vi "dynamic_lights.vi"() -> ()   [LabVIEW 2025]
uses:
  <vilib>/MakerHub/LINX/Public/Peripherals/Digital/Digital Write 1 Chan.vi
  <vilib>/MakerHub/LINX/Public/Peripherals/Digital/Digital Write N Chans.vi
  <vilib>/MakerHub/LINX/Private/Local IO/LinxDigitalWrite.vi
  <vilib>/MakerHub/LINX/Public/Utilities/Check Channel.vi
  <vilib>/MakerHub/LINX/Private/Utilties/Generate Error.vi
  <vilib>/Utility/file.llb/Read Delimited Spreadsheet (DBL).vi
  <vilib>/MakerHub/LINX/Public/Utilities/Open Serial.vi
  <vilib>/MakerHub/LINX/LMH-LINX.lvlib
panel:
  in  "em 2":bool
  in  "em 1":bool
  out "Emergency 2":bool
  out "Emergency 1":bool
  in  "Stop Button":bool
  in  "Stop":bool
  out "Lane 1 Elapsed Time":dbl
  out "Red 2":bool
  out "Orange 2":bool
  out "Green 2":bool
  out "Red 1":bool
  out "Orange 1":bool
  out "Green 1":bool
  out "Lan 2 Elapsed Time":dbl
  out "Lane 2 PCE":dbl
  out "Lane 1 PCE":dbl
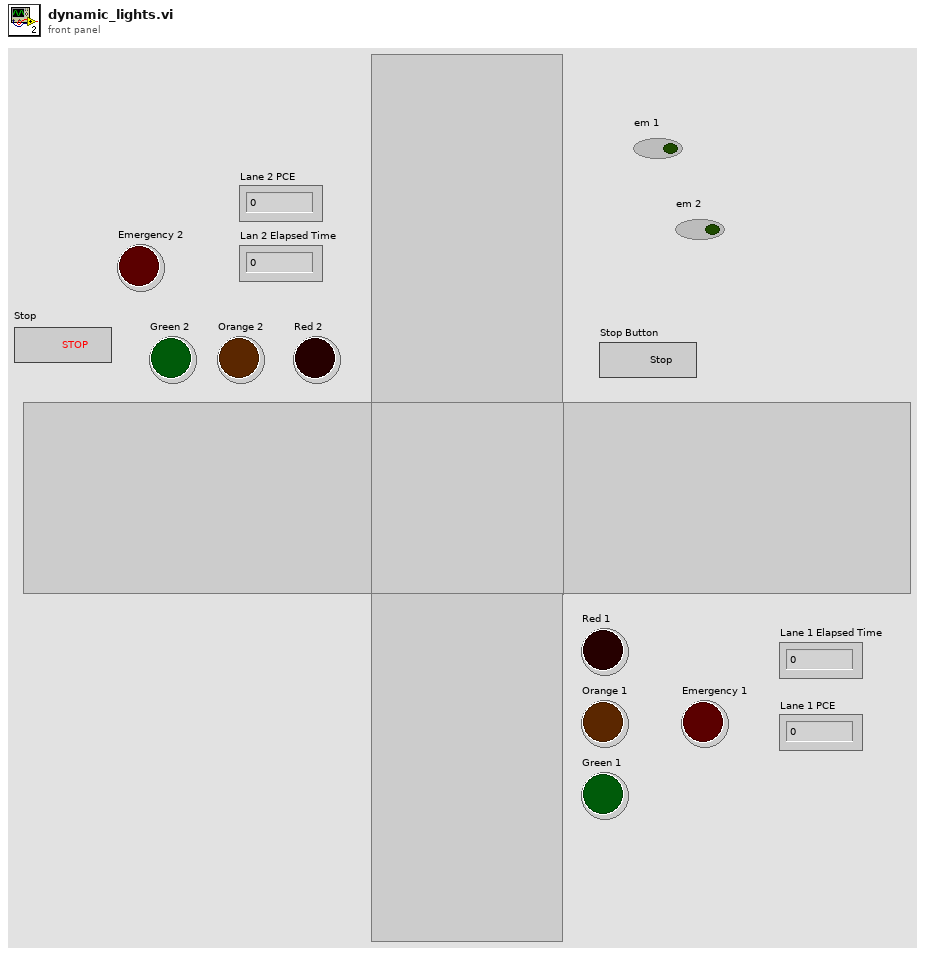
[diagram p1: front panel]
types:
  T1 = typedef "LMH-LINX.lvlib/LINX Ref.ctl" = cluster{"IO":T2, "Interface":T3, "LINX Device Config":T4}
  T2 = typedef "LMH-LINX.lvlib/Platform.ctl" = enum16{"Remote", "Local"}
  T3 = typedef "LMH-LINX.lvlib/Interface.ctl" = enum16{"Serial", "TCP"}
  T4 = typedef "LMH-LINX.lvlib/Device.lvlib/LINX Device Config.ctl" = cluster{"Interface":T3, "COM Port":refnum<visa-resource-name>, "TCP Configuration":T5, "Device Family":u8, "Device ID":u8, "Device Name":string, "TCP Ref":refnum<k5>, "Channels":T6}
  T5 = typedef "LMH-LINX.lvlib/Device.lvlib/TCP Config.ctl" = cluster{"IP Address":string, "Port":u16}
  T6 = typedef "LMH-LINX.lvlib/Channels.ctl" = cluster{"DI":u8[], "DO":u8[], "AI":u8[], "AO":u8[], "PWM":u8[], "QE":u8[], "UART":u8[], "I2C 2":u8[], "SPI":u8[], "CAN":u8[], "Servo":u8[], "AI Ref (V)":dbl, "AI Resolution (Bits)":u8, "AO Ref (V)":dbl, "AO Resolution (Bits)":u8}
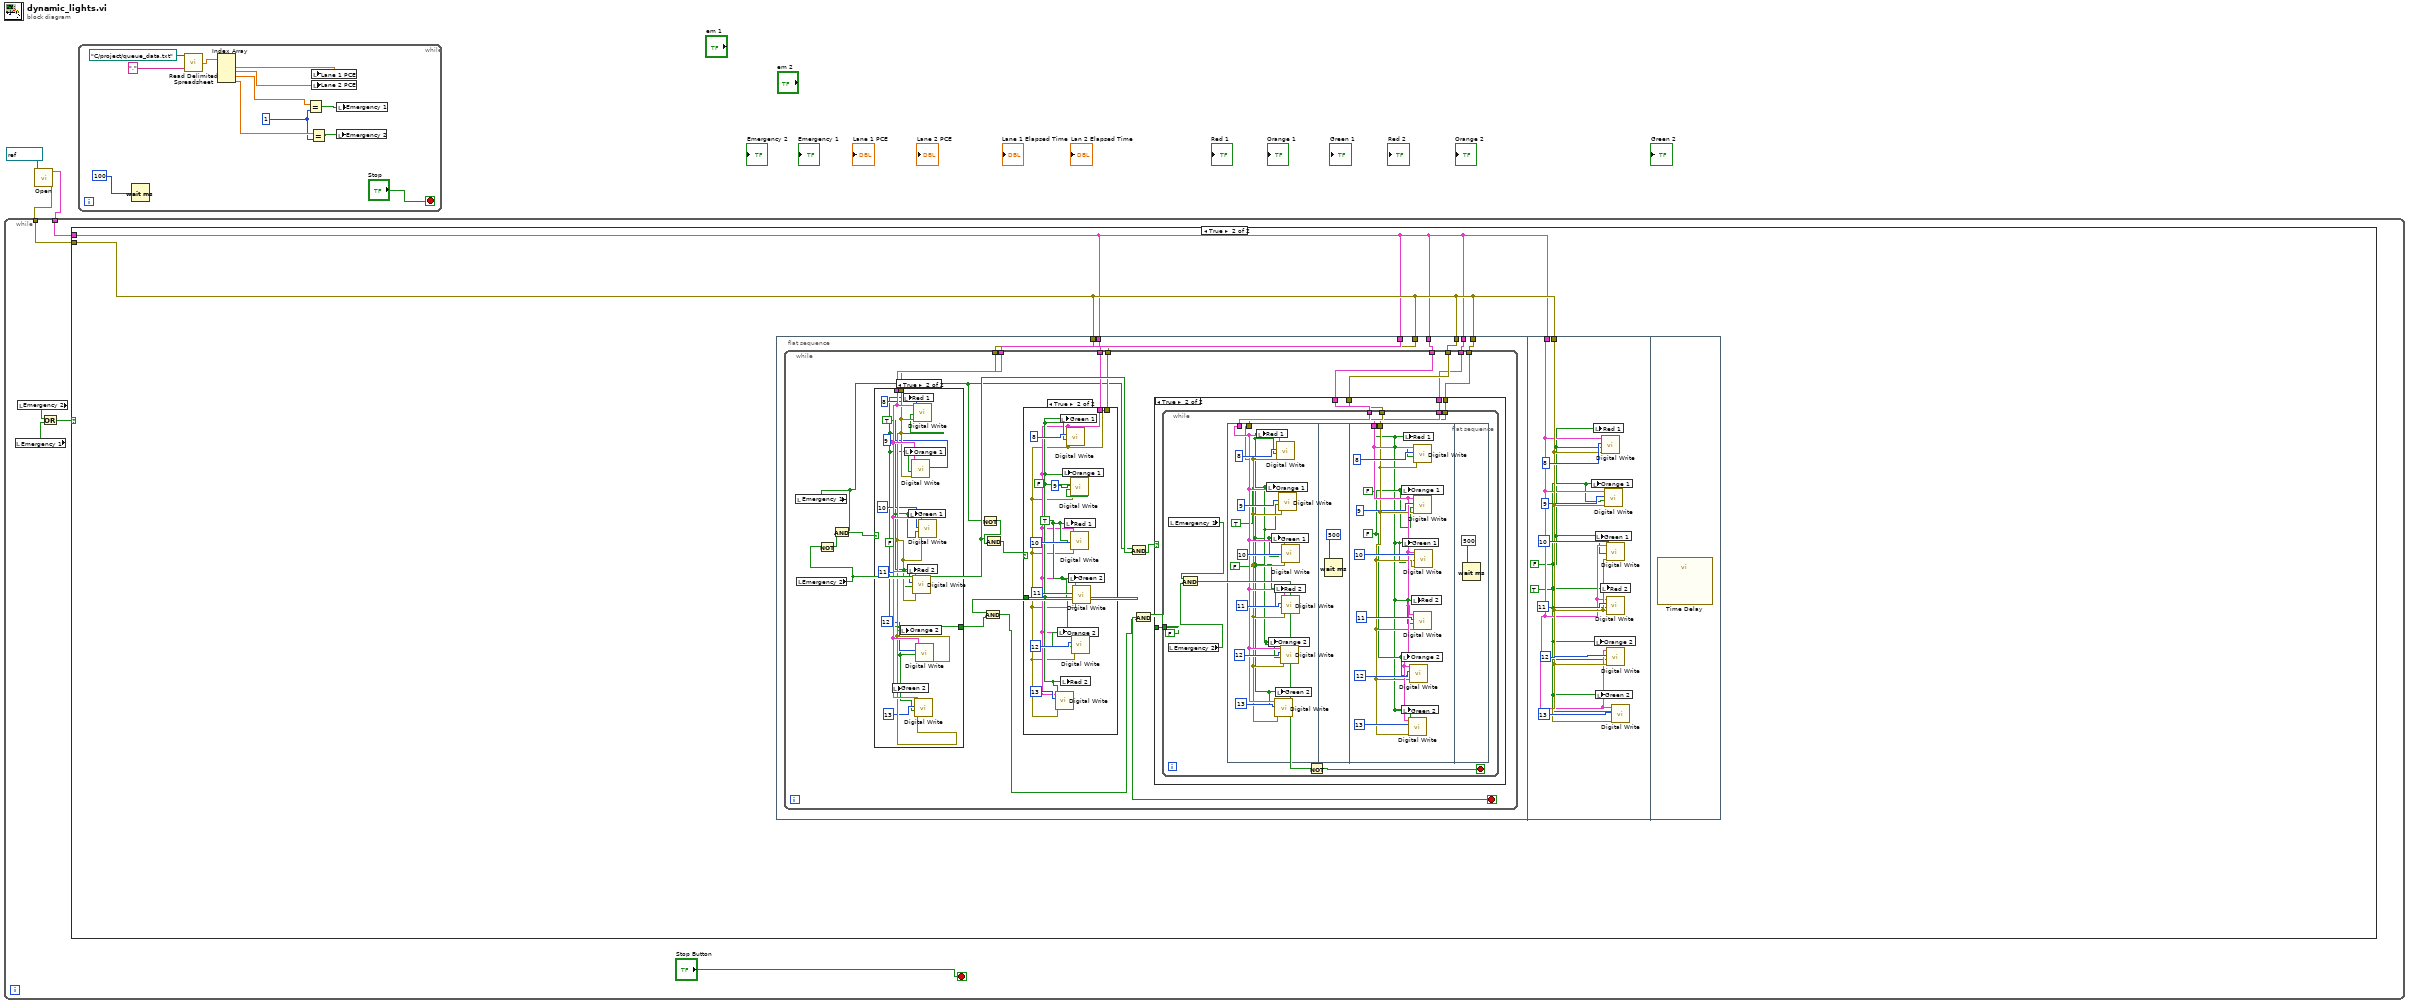
[diagram p0: block diagram]
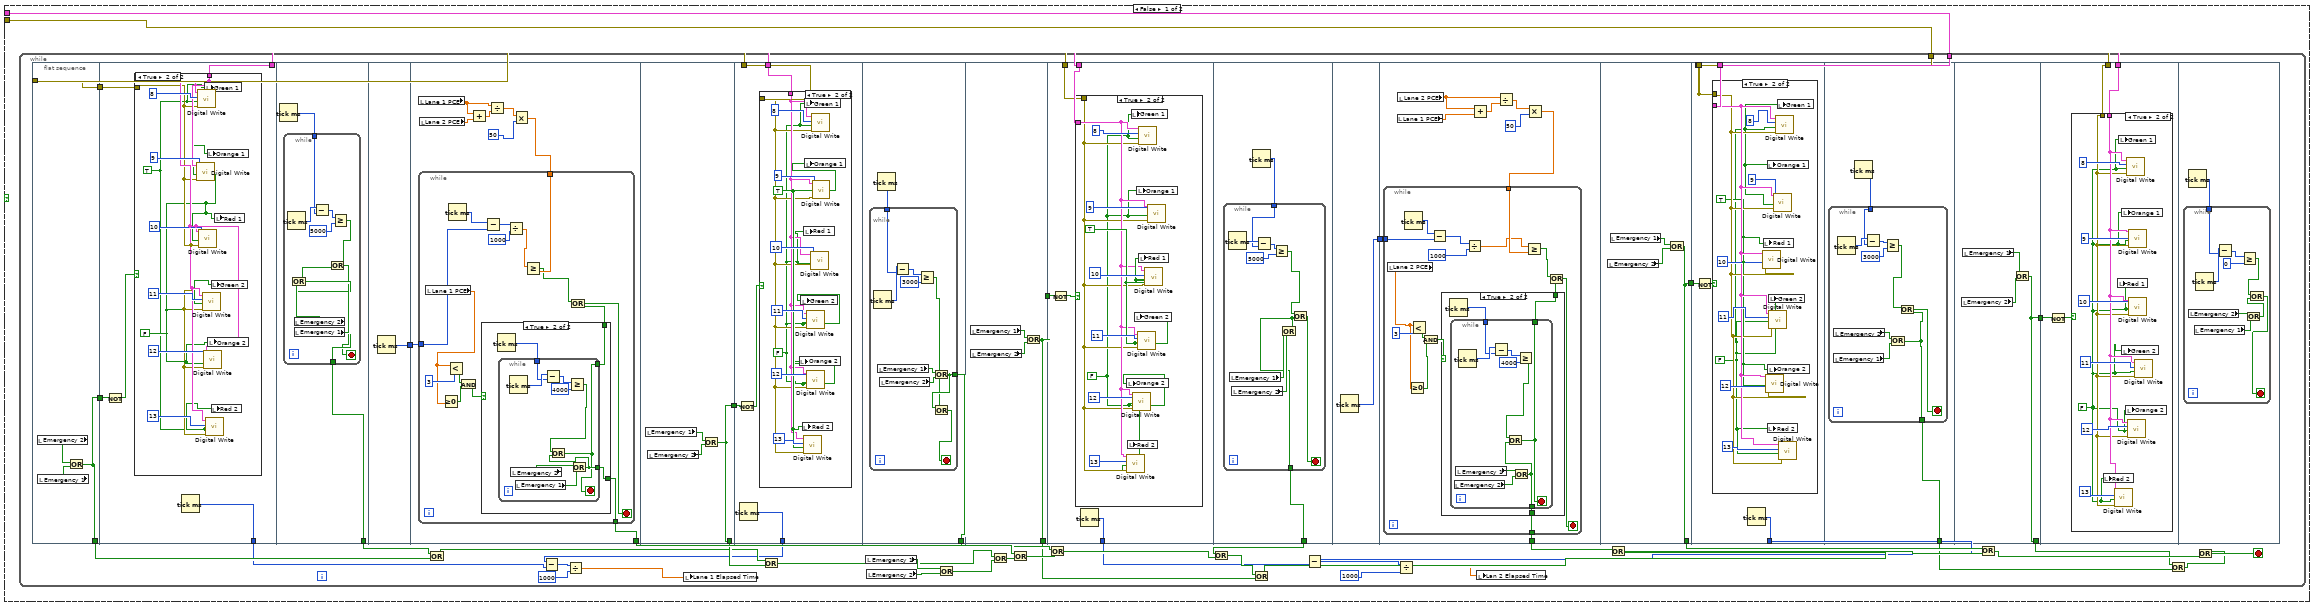
[diagram p2: hidden frame]
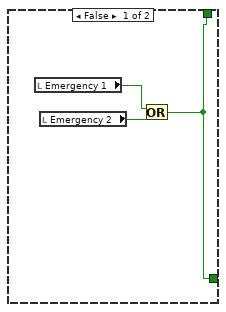
[diagram p4: hidden frame]
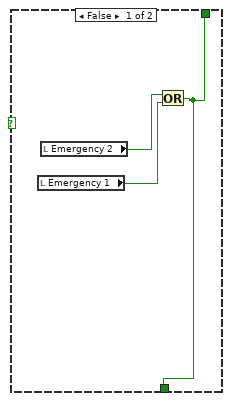
[diagram p7: hidden frame]
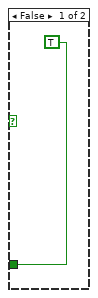
[diagram p10: hidden frame]
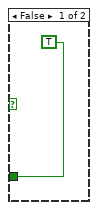
[diagram p11: hidden frame]
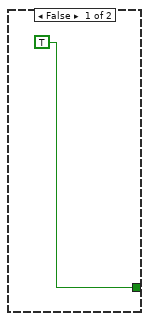
[diagram p12: hidden frame]
diagram:
  n1 = call-poly <vilib>:"Open.vi"("Serial Port"=refnum<visa-resource-name> "COM3") -> ("Error Out"=w1:errorcluster, "LINX Resource"=w2:T1)  [unwired: 8 in, 1 out]
  n2 = while {
    tunnel: w2 -> [w8]
    tunnel: w1 -> [w7]
    stop <- "Stop Button" stop-if-true
    n3 = local read "Emergency 1"() -> (w5:bool)
    n4 = local read "Emergency 2"() -> (w4:bool)
    n5 = Or(x=w4, y=w5) -> (x .or. y?=w6:bool)
    n6 = case shown="True" w6 {
      tunnel: w8 -> [w11 w278]
      tunnel: w7 -> [w10 w279]
      frame False {
        n7 = while {
          tunnel: w11 -> [w54]
          tunnel: w10 -> [w53]
          stop <- w42 stop-if-true
          n8 = flat-sequence {
            tunnel: w53 -> [w60]
            tunnel: [w60] -> w40
            tunnel: [w57] -> w39
            tunnel: [w57] -> w19
            tunnel: w54 -> [w65]
            tunnel: [w63] -> w24
            tunnel: w40 -> [w64]
            tunnel: w19 -> [w61]
            tunnel: [w77] -> w41
            tunnel: [w87] -> w56
            tunnel: w56 -> [w95]
            tunnel: [w88] -> w48
            tunnel: [w126] -> w38
            tunnel: [w126] -> w18
            tunnel: [w133] -> w23
            tunnel: w54 -> [w132]
            tunnel: w53 -> [w131]
            tunnel: w18 -> [w129]
            tunnel: [w145] -> w46
            tunnel: [w155] -> w35
            tunnel: [w155] -> w17
            tunnel: w54 -> [w162]
            tunnel: w53 -> [w161]
            tunnel: [w160] -> w12
            tunnel: w17 -> [w158]
            tunnel: [w174] -> w45
            tunnel: [w184] -> w55
            tunnel: w55 -> [w192]
            tunnel: [w185] -> w43
            tunnel: [w223] -> w32
            tunnel: [w223] -> w16
            tunnel: w54 -> [w230]
            tunnel: [w229] -> _
            tunnel: w53 -> [w229]
            tunnel: [w228] -> w20
            tunnel: w16 -> [w226]
            tunnel: [w242] -> w28
            tunnel: [w252] -> w29
            tunnel: [w252] -> w15
            tunnel: w54 -> [w258]
            tunnel: w53 -> [w257]
            tunnel: w15 -> [w255]
            frame #0 {
              n9 = local read "Emergency 2"() -> (w58:bool)
              n10 = local read "Emergency 1"() -> (w59:bool)
              n11 = Or(x=w58, y=w59) -> (x .or. y?=w57:bool)
            }
            frame #1 {
              n12 = Not(x=w61) -> (.not. x?=w62:bool)
              n13 = case shown="True" w62 {
                tunnel: w65 -> [_ w69]
                tunnel: w64 -> [_ w68]
                frame False {
                }
                frame True {
                  w67 = FALSE
                  w66 = TRUE
                  n14 = call-poly <vilib>:"Digital Write.vi"("Error In"=w68, "Output Value"=w67, "DO Channel"=9, "LINX Resource"=w69) -> ()  [unwired: 6 in, 2 out]
                  n15 = call-poly <vilib>:"Digital Write.vi"("Error In"=w68, "Output Value"=w66, "DO Channel"=8, "LINX Resource"=w69) -> ()  [unwired: 6 in, 2 out]
                  n16 = call-poly <vilib>:"Digital Write.vi"("Error In"=w68, "Output Value"=w67, "DO Channel"=10, "LINX Resource"=w69) -> ()  [unwired: 6 in, 2 out]
                  n17 = call-poly <vilib>:"Digital Write.vi"("Error In"=w68, "Output Value"=w67, "DO Channel"=11, "LINX Resource"=w69) -> ()  [unwired: 6 in, 2 out]
                  n18 = call-poly <vilib>:"Digital Write.vi"("Error In"=w68, "Output Value"=w67, "DO Channel"=12, "LINX Resource"=w69) -> ()  [unwired: 6 in, 2 out]
                  n19 = local write "Green 1"(w66) -> ()
                  n20 = call-poly <vilib>:"Digital Write.vi"("Error In"=w68, "Output Value"=w66, "DO Channel"=13, "LINX Resource"=w69) -> ()  [unwired: 6 in, 2 out]
                  n21 = local write "Orange 1"(w67) -> ()
                  n22 = local write "Orange 2"(w67) -> ()
                  n23 = local write "Green 2"(w67) -> ()
                  n24 = local write "Red 2"(w66) -> ()
                  n25 = local write "Red 1"(w67) -> ()
                }
              }
              n26 = Tick Count (ms)() -> (millisecond timer value=w63:u32)
            }
            frame #2 {
              n27 = Tick Count (ms)() -> (millisecond timer value=w76:u32)
              n28 = while {
                tunnel: [w84] -> w77
                tunnel: w76 -> [w79]
                stop <- w83 stop-if-true
                n29 = Tick Count (ms)() -> (millisecond timer value=w82:u32)
                n30 = local read "Emergency 2"() -> (w86:bool)
                n31 = local read "Emergency 1"() -> (w85:bool)
                n32 = Or(x=w86, y=w85) -> (x .or. y?=w84:bool)
                n33 = Subtract(x=w82, y=w79) -> (x-y=w81:u32)
                n34 = Greater Or Equal?(x=w81, y=5000) -> (x >= y?=w78:bool)
                n35 = Or(x=w78, y=w84) -> (x .or. y?=w83:bool)
              }
            }
            frame #3 {
              n36 = Tick Count (ms)() -> (millisecond timer value=w87:u32)
            }
            frame #4 {
              n37 = local read "Lane 1 PCE"() -> (w92:dbl)
              n38 = local read "Lane 2 PCE"() -> (w94:dbl)
              n39 = Add(x=w92, y=w94) -> (x+y=w93:dbl)
              n40 = Divide(x=w92, y=w93) -> (x/y=w90:dbl)
              n41 = Multiply(x=w90, y=50) -> (x*y=w89:dbl)
              n42 = while {
                tunnel: w95 -> [w109]
                tunnel: w89 -> [w105]
                tunnel: [w99] -> w88
                stop <- w100 stop-if-true
                n43 = local read "Lane 1 PCE"() -> (w97:dbl)
                n44 = Greater Or Equal To 0?(x=w97) -> (x >= 0?=w96:bool)
                n45 = Less?(x=w97, y=3) -> (x < y?=w103:bool)
                n46 = Tick Count (ms)() -> (millisecond timer value=w110:u32)
                n47 = And(x=w103, y=w96) -> (x .and. y?=w102:bool)
                n48 = case shown="True" w102 {
                  tunnel: [w111 w115] -> w101
                  tunnel: [w111 w116] -> w99
                  frame False {
                    n49 = local read "Emergency 1"() -> (w113:bool)
                    n50 = local read "Emergency 2"() -> (w112:bool)
                    n51 = Or(x=w113, y=w112) -> (x .or. y?=w111:bool)
                  }
                  frame True {
                    n52 = Tick Count (ms)() -> (millisecond timer value=w114:u32)
                    n53 = while {
                      tunnel: [w123] -> w116
                      tunnel: [w122] -> w115
                      tunnel: w114 -> [w117]
                      stop <- w122 stop-if-true
                      n54 = Tick Count (ms)() -> (millisecond timer value=w121:u32)
                      n55 = local read "Emergency 2"() -> (w124:bool)
                      n56 = local read "Emergency 1"() -> (w125:bool)
                      n57 = Subtract(x=w121, y=w117) -> (x-y=w120:u32)
                      n58 = Greater Or Equal?(x=w120, y=4000) -> (x >= y?=w118:bool)
                      n59 = Or(x=w124, y=w125) -> (x .or. y?=w123:bool)
                      n60 = Or(x=w118, y=w123) -> (x .or. y?=w122:bool)
                    }
                  }
                }
                n61 = Subtract(x=w110, y=w109) -> (x-y=w107:u32)
                n62 = Divide(x=w107, y=1000) -> (x/y=w106:dbl)
                n63 = Greater Or Equal?(x=w106, y=w105) -> (x >= y?=w98:bool)
                n64 = Or(x=w98, y=w101) -> (x .or. y?=w100:bool)
              }
            }
            frame #5 {
              n65 = local read "Emergency 1"() -> (w128:bool)
              n66 = local read "Emergency 2"() -> (w127:bool)
              n67 = Or(x=w128, y=w127) -> (x .or. y?=w126:bool)
            }
            frame #6 {
              n68 = Not(x=w129) -> (.not. x?=w130:bool)
              n69 = Tick Count (ms)() -> (millisecond timer value=w133:u32)
              n70 = case shown="True" w130 {
                tunnel: w132 -> [_ w136]
                tunnel: w131 -> [_ w135]
                frame False {
                }
                frame True {
                  w134 = FALSE
                  w137 = TRUE
                  n71 = local write "Orange 2"(w134) -> ()
                  n72 = local write "Green 2"(w134) -> ()
                  n73 = local write "Red 2"(w137) -> ()
                  n74 = call-poly <vilib>:"Digital Write.vi"("Error In"=w135, "Output Value"=w137, "DO Channel"=13, "LINX Resource"=w136) -> ()  [unwired: 6 in, 2 out]
                  n75 = local write "Red 1"(w134) -> ()
                  n76 = local write "Green 1"(w134) -> ()
                  n77 = local write "Orange 1"(w137) -> ()
                  n78 = call-poly <vilib>:"Digital Write.vi"("Error In"=w135, "Output Value"=w134, "DO Channel"=11, "LINX Resource"=w136) -> ()  [unwired: 6 in, 2 out]
                  n79 = call-poly <vilib>:"Digital Write.vi"("Error In"=w135, "Output Value"=w134, "DO Channel"=12, "LINX Resource"=w136) -> ()  [unwired: 6 in, 2 out]
                  n80 = call-poly <vilib>:"Digital Write.vi"("Error In"=w135, "Output Value"=w134, "DO Channel"=10, "LINX Resource"=w136) -> ()  [unwired: 6 in, 2 out]
                  n81 = call-poly <vilib>:"Digital Write.vi"("Error In"=w135, "Output Value"=w134, "DO Channel"=8, "LINX Resource"=w136) -> ()  [unwired: 6 in, 2 out]
                  n82 = call-poly <vilib>:"Digital Write.vi"("Error In"=w135, "Output Value"=w137, "DO Channel"=9, "LINX Resource"=w136) -> ()  [unwired: 6 in, 2 out]
                }
              }
            }
            frame #7 {
              n83 = Tick Count (ms)() -> (millisecond timer value=w144:u32)
              n84 = while {
                tunnel: [w151] -> w145
                tunnel: w144 -> [w146]
                stop <- w152 stop-if-true
                n85 = Tick Count (ms)() -> (millisecond timer value=w150:u32)
                n86 = local read "Emergency 1"() -> (w154:bool)
                n87 = local read "Emergency 2"() -> (w153:bool)
                n88 = Subtract(x=w150, y=w146) -> (x-y=w149:u32)
                n89 = Greater Or Equal?(x=w149, y=3000) -> (x >= y?=w147:bool)
                n90 = Or(x=w154, y=w153) -> (x .or. y?=w151:bool)
                n91 = Or(x=w151, y=w147) -> (x .or. y?=w152:bool)
              }
            }
            frame #8 {
              n92 = local read "Emergency 1"() -> (w156:bool)
              n93 = local read "Emergency 2"() -> (w157:bool)
              n94 = Or(x=w156, y=w157) -> (x .or. y?=w155:bool)
            }
            frame #9 {
              n95 = Not(x=w158) -> (.not. x?=w159:bool)
              n96 = case shown="True" w159 {
                tunnel: w162 -> [_ w165]
                tunnel: w161 -> [_ w164]
                frame False {
                }
                frame True {
                  w163 = FALSE
                  w166 = TRUE
                  n97 = call-poly <vilib>:"Digital Write.vi"("Error In"=w164, "Output Value"=w163, "DO Channel"=13, "LINX Resource"=w165) -> ()  [unwired: 6 in, 2 out]
                  n98 = local write "Orange 2"(w163) -> ()
                  n99 = local write "Red 2"(w163) -> ()
                  n100 = local write "Green 1"(w163) -> ()
                  n101 = call-poly <vilib>:"Digital Write.vi"("Error In"=w164, "Output Value"=w163, "DO Channel"=12, "LINX Resource"=w165) -> ()  [unwired: 6 in, 2 out]
                  n102 = local write "Green 2"(w166) -> ()
                  n103 = local write "Orange 1"(w163) -> ()
                  n104 = call-poly <vilib>:"Digital Write.vi"("Error In"=w164, "Output Value"=w166, "DO Channel"=11, "LINX Resource"=w165) -> ()  [unwired: 6 in, 2 out]
                  n105 = call-poly <vilib>:"Digital Write.vi"("Error In"=w164, "Output Value"=w163, "DO Channel"=8, "LINX Resource"=w165) -> ()  [unwired: 6 in, 2 out]
                  n106 = local write "Red 1"(w166) -> ()
                  n107 = call-poly <vilib>:"Digital Write.vi"("Error In"=w164, "Output Value"=w166, "DO Channel"=10, "LINX Resource"=w165) -> ()  [unwired: 6 in, 2 out]
                  n108 = call-poly <vilib>:"Digital Write.vi"("Error In"=w164, "Output Value"=w163, "DO Channel"=9, "LINX Resource"=w165) -> ()  [unwired: 6 in, 2 out]
                }
              }
              n109 = Tick Count (ms)() -> (millisecond timer value=w160:u32)
            }
            frame #10 {
              n110 = Tick Count (ms)() -> (millisecond timer value=w173:u32)
              n111 = while {
                tunnel: [w180] -> w174
                tunnel: w173 -> [w175]
                stop <- w181 stop-if-true
                n112 = Tick Count (ms)() -> (millisecond timer value=w179:u32)
                n113 = local read "Emergency 1"() -> (w183:bool)
                n114 = local read "Emergency 2"() -> (w182:bool)
                n115 = Subtract(x=w179, y=w175) -> (x-y=w178:u32)
                n116 = Greater Or Equal?(x=w178, y=5000) -> (x >= y?=w176:bool)
                n117 = Or(x=w183, y=w182) -> (x .or. y?=w180:bool)
                n118 = Or(x=w176, y=w180) -> (x .or. y?=w181:bool)
              }
            }
            frame #11 {
              n119 = Tick Count (ms)() -> (millisecond timer value=w184:u32)
            }
            frame #12 {
              n120 = local read "Lane 1 PCE"() -> (w191:dbl)
              n121 = local read "Lane 2 PCE"() -> (w189:dbl)
              n122 = Add(x=w189, y=w191) -> (x+y=w190:dbl)
              n123 = Divide(x=w189, y=w190) -> (x/y=w188:dbl)
              n124 = Multiply(x=w188, y=50) -> (x*y=w186:dbl)
              n125 = while {
                tunnel: w192 -> [w206]
                tunnel: w186 -> [w203]
                tunnel: [w196] -> w185
                stop <- w197 stop-if-true
                n126 = local read "Lane 2 PCE"() -> (w195:dbl)
                n127 = Tick Count (ms)() -> (millisecond timer value=w207:u32)
                n128 = Greater Or Equal To 0?(x=w195) -> (x >= 0?=w194:bool)
                n129 = Less?(x=w195, y=3) -> (x < y?=w200:bool)
                n130 = And(x=w200, y=w194) -> (x .and. y?=w199:bool)
                n131 = Subtract(x=w207, y=w206) -> (x-y=w204:u32)
                n132 = case shown="True" w199 {
                  tunnel: [w208 w213] -> w198
                  tunnel: [w208 w212] -> w196
                  frame False {
                    n133 = local read "Emergency 1"() -> (w209:bool)
                    n134 = local read "Emergency 2"() -> (w210:bool)
                    n135 = Or(x=w210, y=w209) -> (x .or. y?=w208:bool)
                  }
                  frame True {
                    n136 = Tick Count (ms)() -> (millisecond timer value=w211:u32)
                    n137 = while {
                      tunnel: [w220] -> w213
                      tunnel: [w219] -> w212
                      tunnel: w211 -> [w214]
                      stop <- w220 stop-if-true
                      n138 = local read "Emergency 2"() -> (w221:bool)
                      n139 = local read "Emergency 1"() -> (w222:bool)
                      n140 = Tick Count (ms)() -> (millisecond timer value=w218:u32)
                      n141 = Subtract(x=w218, y=w214) -> (x-y=w217:u32)
                      n142 = Or(x=w222, y=w221) -> (x .or. y?=w219:bool)
                      n143 = Greater Or Equal?(x=w217, y=4000) -> (x >= y?=w215:bool)
                      n144 = Or(x=w215, y=w219) -> (x .or. y?=w220:bool)
                    }
                  }
                }
                n145 = Divide(x=w204, y=1000) -> (x/y=w202:dbl)
                n146 = Greater Or Equal?(x=w202, y=w203) -> (x >= y?=w193:bool)
                n147 = Or(x=w193, y=w198) -> (x .or. y?=w197:bool)
              }
            }
            frame #13 {
              n148 = local read "Emergency 2"() -> (w224:bool)
              n149 = local read "Emergency 1"() -> (w225:bool)
              n150 = Or(x=w225, y=w224) -> (x .or. y?=w223:bool)
            }
            frame #14 {
              n151 = Not(x=w226) -> (.not. x?=w227:bool)
              n152 = case shown="True" w227 {
                tunnel: w230 -> [_ w234]
                tunnel: w229 -> [_ w233]
                frame False {
                }
                frame True {
                  w231 = FALSE
                  w232 = TRUE
                  n153 = call-poly <vilib>:"Digital Write.vi"("Error In"=w233, "Output Value"=w232, "DO Channel"=10, "LINX Resource"=w234) -> ()  [unwired: 6 in, 2 out]
                  n154 = local write "Red 1"(w232) -> ()
                  n155 = call-poly <vilib>:"Digital Write.vi"("Error In"=w233, "Output Value"=w232, "DO Channel"=12, "LINX Resource"=w234) -> ()  [unwired: 6 in, 2 out]
                  n156 = local write "Orange 1"(w231) -> ()
                  n157 = local write "Red 2"(w231) -> ()
                  n158 = local write "Orange 2"(w232) -> ()
                  n159 = local write "Green 2"(w231) -> ()
                  n160 = call-poly <vilib>:"Digital Write.vi"("Error In"=w233, "Output Value"=w231, "DO Channel"=11, "LINX Resource"=w234) -> ()  [unwired: 6 in, 2 out]
                  n161 = call-poly <vilib>:"Digital Write.vi"("Error In"=w233, "Output Value"=w231, "DO Channel"=9, "LINX Resource"=w234) -> ()  [unwired: 6 in, 2 out]
                  n162 = call-poly <vilib>:"Digital Write.vi"("Error In"=w233, "Output Value"=w231, "DO Channel"=8, "LINX Resource"=w234) -> ()  [unwired: 6 in, 2 out]
                  n163 = local write "Green 1"(w231) -> ()
                  n164 = call-poly <vilib>:"Digital Write.vi"("Error In"=w233, "Output Value"=w231, "DO Channel"=13, "LINX Resource"=w234) -> ()  [unwired: 6 in, 2 out]
                }
              }
              n165 = Tick Count (ms)() -> (millisecond timer value=w228:u32)
            }
            frame #15 {
              n166 = Tick Count (ms)() -> (millisecond timer value=w241:u32)
              n167 = while {
                tunnel: [w248] -> w242
                tunnel: w241 -> [w246]
                stop <- w249 stop-if-true
                n168 = local read "Emergency 1"() -> (w250:bool)
                n169 = local read "Emergency 2"() -> (w251:bool)
                n170 = Tick Count (ms)() -> (millisecond timer value=w247:u32)
                n171 = Subtract(x=w247, y=w246) -> (x-y=w245:u32)
                n172 = Greater Or Equal?(x=w245, y=3000) -> (x >= y?=w243:bool)
                n173 = Or(x=w251, y=w250) -> (x .or. y?=w248:bool)
                n174 = Or(x=w243, y=w248) -> (x .or. y?=w249:bool)
              }
            }
            frame #16 {
              n175 = local read "Emergency 2"() -> (w253:bool)
              n176 = local read "Emergency 1"() -> (w254:bool)
              n177 = Or(x=w254, y=w253) -> (x .or. y?=w252:bool)
            }
            frame #17 {
              n178 = Not(x=w255) -> (.not. x?=w256:bool)
              n179 = case shown="True" w256 {
                tunnel: w258 -> [_ w261]
                tunnel: w257 -> [_ w260]
                frame False {
                }
                frame True {
                  w259 = FALSE
                  n180 = local write "Red 2"(w259) -> ()
                  n181 = call-poly <vilib>:"Digital Write.vi"("Error In"=w260, "Output Value"=w259, "DO Channel"=13, "LINX Resource"=w261) -> ()  [unwired: 6 in, 2 out]
                  n182 = local write "Red 1"(w259) -> ()
                  n183 = local write "Green 1"(w259) -> ()
                  n184 = local write "Orange 1"(w259) -> ()
                  n185 = local write "Green 2"(w259) -> ()
                  n186 = local write "Orange 2"(w259) -> ()
                  n187 = call-poly <vilib>:"Digital Write.vi"("Error In"=w260, "Output Value"=w259, "DO Channel"=8, "LINX Resource"=w261) -> ()  [unwired: 6 in, 2 out]
                  n188 = call-poly <vilib>:"Digital Write.vi"("Error In"=w260, "Output Value"=w259, "DO Channel"=12, "LINX Resource"=w261) -> ()  [unwired: 6 in, 2 out]
                  n189 = call-poly <vilib>:"Digital Write.vi"("Error In"=w260, "Output Value"=w259, "DO Channel"=9, "LINX Resource"=w261) -> ()  [unwired: 6 in, 2 out]
                  n190 = call-poly <vilib>:"Digital Write.vi"("Error In"=w260, "Output Value"=w259, "DO Channel"=10, "LINX Resource"=w261) -> ()  [unwired: 6 in, 2 out]
                  n191 = call-poly <vilib>:"Digital Write.vi"("Error In"=w260, "Output Value"=w259, "DO Channel"=11, "LINX Resource"=w261) -> ()  [unwired: 6 in, 2 out]
                }
              }
            }
            frame #18 {
              n192 = Tick Count (ms)() -> (millisecond timer value=w268:u32)
              n193 = while {
                tunnel: w268 -> [w274]
                stop <- w269 stop-if-true
                n194 = local read "Emergency 2"() -> (w272:bool)
                n195 = local read "Emergency 1"() -> (w273:bool)
                n196 = Tick Count (ms)() -> (millisecond timer value=w277:u32)
                n197 = Subtract(x=w277, y=w274) -> (x-y=w276:u32)
                n198 = Greater Or Equal?(x=w276, y=0) -> (x >= y?=w270:bool)
                n199 = Or(x=w272, y=w273) -> (x .or. y?=w271:bool)
                n200 = Or(x=w270, y=w271) -> (x .or. y?=w269:bool)
              }
            }
          }
          n201 = Or(x=w41, y=w39) -> (x .or. y?=w37:bool)
          n202 = Subtract(x=w23, y=w24) -> (x-y=w26:u32)
          n203 = Divide(x=w26, y=1000) -> (x/y=w14:dbl)
          n204 = local write "Lane 1 Elapsed Time"(w14) -> ()
          n205 = Or(x=w37, y=w38) -> (x .or. y?=w36:bool)
          n206 = local read "Emergency 1"() -> (w52:bool)
          n207 = local read "Emergency 2"() -> (w51:bool)
          n208 = Or(x=w52, y=w51) -> (x .or. y?=w50:bool)
          n209 = Or(x=w36, y=w50) -> (x .or. y?=w49:bool)
          n210 = Or(x=w48, y=w49) -> (x .or. y?=w47:bool)
          n211 = Or(x=w46, y=w47) -> (x .or. y?=w44:bool)
          n212 = Or(x=w45, y=w44) -> (x .or. y?=w34:bool)
          n213 = Or(x=w34, y=w35) -> (x .or. y?=w33:bool)
          n214 = Subtract(x=w20, y=w12) -> (x-y=w22:u32)
          n215 = Divide(x=w22, y=1000) -> (x/y=w13:dbl)
          n216 = local write "Lan 2 Elapsed Time"(w13) -> ()
          n217 = Or(x=w43, y=w33) -> (x .or. y?=w31:bool)
          n218 = Or(x=w32, y=w31) -> (x .or. y?=w30:bool)
          n219 = Or(x=w29, y=w28) -> (x .or. y?=w27:bool)
          n220 = Or(x=w27, y=w30) -> (x .or. y?=w42:bool)
        }
      }
      frame True {
        n221 = flat-sequence {
          tunnel: w278 -> [w287]
          tunnel: w279 -> [w286]
          tunnel: w278 -> [w285]
          tunnel: w279 -> [w284]
          tunnel: w278 -> [w283]
          tunnel: w279 -> [w282]
          tunnel: w278 -> [w281]
          tunnel: w279 -> [w280]
          tunnel: w279 -> [w370]
          tunnel: w278 -> [w369]
          frame #0 {
            n222 = while {
              tunnel: w287 -> [w296]
              tunnel: w286 -> [w295]
              tunnel: w285 -> [w294]
              tunnel: w284 -> [w293]
              tunnel: w283 -> [w292]
              tunnel: w282 -> [w291]
              tunnel: w281 -> [w290]
              tunnel: w280 -> [w289]
              stop <- w299 stop-if-true
              n223 = local read "Emergency 1"() -> (w288:bool)
              n224 = local read "Emergency 2"() -> (w302:bool)
              n225 = Not(x=w302) -> (.not. x?=w304:bool)
              n226 = And(x=w288, y=w304) -> (x .and. y?=w303:bool)
              n227 = case shown="True" w303 {
                tunnel: [TRUE w357] -> w300
                tunnel: w294 -> [_ w366]
                tunnel: w293 -> [_ w365]
                frame False {
                }
                frame True {
                  w357 = FALSE
                  w358 = TRUE
                  n228 = local write "Green 2"(w357) -> ()
                  n229 = local write "Orange 2"(w357) -> ()
                  n230 = local write "Red 1"(w357) -> ()
                  n231 = local write "Orange 1"(w357) -> ()
                  n232 = local write "Red 2"(w358) -> ()
                  n233 = local write "Green 1"(w358) -> ()
                  n234 = call-poly <vilib>:"Digital Write.vi"("Error In"=w365, "Output Value"=w357, "DO Channel"=9, "LINX Resource"=w366) -> ()  [unwired: 6 in, 2 out]
                  n235 = call-poly <vilib>:"Digital Write.vi"("Error In"=w365, "Output Value"=w358, "DO Channel"=11, "LINX Resource"=w366) -> ()  [unwired: 6 in, 2 out]
                  n236 = call-poly <vilib>:"Digital Write.vi"("Error In"=w365, "Output Value"=w357, "DO Channel"=8, "LINX Resource"=w366) -> ()  [unwired: 6 in, 2 out]
                  n237 = call-poly <vilib>:"Digital Write.vi"("Error In"=w365, "Output Value"=w357, "DO Channel"=13, "LINX Resource"=w366) -> ()  [unwired: 6 in, 2 out]
                  n238 = call-poly <vilib>:"Digital Write.vi"("Error In"=w365, "Output Value"=w357, "DO Channel"=12, "LINX Resource"=w366) -> ()  [unwired: 6 in, 2 out]
                  n239 = call-poly <vilib>:"Digital Write.vi"("Error In"=w365, "Output Value"=w358, "DO Channel"=10, "LINX Resource"=w366) -> ()  [unwired: 6 in, 2 out]
                }
              }
              n240 = Not(x=w288) -> (.not. x?=w307:bool)
              n241 = And(x=w302, y=w307) -> (x .and. y?=w306:bool)
              n242 = case shown="True" w306 {
                tunnel: [TRUE w349] -> w301
                tunnel: w296 -> [_ w347]
                tunnel: w295 -> [_ w346]
                frame False {
                }
                frame True {
                  w349 = FALSE
                  w350 = TRUE
                  n243 = call-poly <vilib>:"Digital Write.vi"("Error In"=w346, "Output Value"=w349, "DO Channel"=13, "LINX Resource"=w347) -> ()  [unwired: 6 in, 2 out]
                  n244 = local write "Orange 2"(w349) -> ()
                  n245 = local write "Green 1"(w349) -> ()
                  n246 = local write "Red 2"(w349) -> ()
                  n247 = local write "Orange 1"(w349) -> ()
                  n248 = local write "Red 1"(w350) -> ()
                  n249 = call-poly <vilib>:"Digital Write.vi"("Error In"=w346, "Output Value"=w349, "DO Channel"=8, "LINX Resource"=w347) -> ()  [unwired: 6 in, 2 out]
                  n250 = local write "Green 2"(w350) -> ()
                  n251 = call-poly <vilib>:"Digital Write.vi"("Error In"=w346, "Output Value"=w349, "DO Channel"=9, "LINX Resource"=w347) -> ()  [unwired: 6 in, 2 out]
                  n252 = call-poly <vilib>:"Digital Write.vi"("Error In"=w346, "Output Value"=w350, "DO Channel"=10, "LINX Resource"=w347) -> ()  [unwired: 6 in, 2 out]
                  n253 = call-poly <vilib>:"Digital Write.vi"("Error In"=w346, "Output Value"=w349, "DO Channel"=12, "LINX Resource"=w347) -> ()  [unwired: 6 in, 2 out]
                  n254 = call-poly <vilib>:"Digital Write.vi"("Error In"=w346, "Output Value"=w350, "DO Channel"=11, "LINX Resource"=w347) -> ()  [unwired: 6 in, 2 out]
                }
              }
              n255 = And(x=w301, y=w300) -> (x .and. y?=w297:bool)
              n256 = And(x=w288, y=w302) -> (x .and. y?=w305:bool)
              n257 = case shown="True" w305 {
                tunnel: [TRUE w309] -> w298
                tunnel: w292 -> [_ w313]
                tunnel: w291 -> [_ w312]
                tunnel: w290 -> [_ w311]
                tunnel: w289 -> [_ w310]
                frame False {
                }
                frame True {
                  n258 = while {
                    tunnel: w313 -> [w318]
                    tunnel: w312 -> [w317]
                    tunnel: w311 -> [w316]
                    tunnel: w310 -> [w315]
                    tunnel: [FALSE] -> w309
                    stop <- w321 stop-if-true
                    n259 = local read "Emergency 2"() -> (w319:bool)
                    n260 = local read "Emergency 1"() -> (w320:bool)
                    n261 = And(x=w320, y=w319) -> (x .and. y?=w322:bool)
                    n262 = flat-sequence {
                      tunnel: w318 -> [w326]
                      tunnel: w317 -> [w325]
                      tunnel: w316 -> [w337]
                      tunnel: w315 -> [w336]
                      frame #0 {
                        w323 = FALSE
                        w324 = TRUE
                        n263 = local write "Red 1"(w323) -> ()
                        n264 = local write "Orange 1"(w324) -> ()
                        n265 = local write "Orange 2"(w324) -> ()
                        n266 = local write "Green 1"(w323) -> ()
                        n267 = local write "Red 2"(w323) -> ()
                        n268 = call-poly <vilib>:"Digital Write.vi"("Error In"=w325, "Output Value"=w323, "DO Channel"=13, "LINX Resource"=w326) -> ()  [unwired: 6 in, 2 out]
                        n269 = local write "Green 2"(w323) -> ()
                        n270 = call-poly <vilib>:"Digital Write.vi"("Error In"=w325, "Output Value"=w323, "DO Channel"=8, "LINX Resource"=w326) -> ()  [unwired: 6 in, 2 out]
                        n271 = call-poly <vilib>:"Digital Write.vi"("Error In"=w325, "Output Value"=w324, "DO Channel"=9, "LINX Resource"=w326) -> ()  [unwired: 6 in, 2 out]
                        n272 = call-poly <vilib>:"Digital Write.vi"("Error In"=w325, "Output Value"=w324, "DO Channel"=12, "LINX Resource"=w326) -> ()  [unwired: 6 in, 2 out]
                        n273 = call-poly <vilib>:"Digital Write.vi"("Error In"=w325, "Output Value"=w323, "DO Channel"=10, "LINX Resource"=w326) -> ()  [unwired: 6 in, 2 out]
                        n274 = call-poly <vilib>:"Digital Write.vi"("Error In"=w325, "Output Value"=w323, "DO Channel"=11, "LINX Resource"=w326) -> ()  [unwired: 6 in, 2 out]
                      }
                      frame #1 {
                        n275 = Wait (ms)(milliseconds to wait=500) -> ()  [unwired: 1 out]
                      }
                      frame #2 {
                        w334 = FALSE
                        w335 = FALSE
                        n276 = local write "Orange 2"(w335) -> ()
                        n277 = local write "Orange 1"(w335) -> ()
                        n278 = local write "Green 2"(w334) -> ()
                        n279 = local write "Green 1"(w334) -> ()
                        n280 = local write "Red 1"(w334) -> ()
                        n281 = call-poly <vilib>:"Digital Write.vi"("Error In"=w336, "Output Value"=w334, "DO Channel"=13, "LINX Resource"=w337) -> ()  [unwired: 6 in, 2 out]
                        n282 = call-poly <vilib>:"Digital Write.vi"("Error In"=w336, "Output Value"=w335, "DO Channel"=12, "LINX Resource"=w337) -> ()  [unwired: 6 in, 2 out]
                        n283 = local write "Red 2"(w334) -> ()
                        n284 = call-poly <vilib>:"Digital Write.vi"("Error In"=w336, "Output Value"=w334, "DO Channel"=8, "LINX Resource"=w337) -> ()  [unwired: 6 in, 2 out]
                        n285 = call-poly <vilib>:"Digital Write.vi"("Error In"=w336, "Output Value"=w335, "DO Channel"=9, "LINX Resource"=w337) -> ()  [unwired: 6 in, 2 out]
                        n286 = call-poly <vilib>:"Digital Write.vi"("Error In"=w336, "Output Value"=w334, "DO Channel"=11, "LINX Resource"=w337) -> ()  [unwired: 6 in, 2 out]
                        n287 = call-poly <vilib>:"Digital Write.vi"("Error In"=w336, "Output Value"=w334, "DO Channel"=10, "LINX Resource"=w337) -> ()  [unwired: 6 in, 2 out]
                      }
                      frame #3 {
                        n288 = Wait (ms)(milliseconds to wait=500) -> ()  [unwired: 1 out]
                      }
                    }
                    n289 = Not(x=w322) -> (.not. x?=w321:bool)
                  }
                }
              }
              n290 = And(x=w298, y=w297) -> (x .and. y?=w299:bool)
            }
          }
          frame #1 {
            w367 = FALSE
            w368 = TRUE
            n291 = local write "Orange 1"(w368) -> ()
            n292 = local write "Red 1"(w367) -> ()
            n293 = local write "Orange 2"(w368) -> ()
            n294 = local write "Green 1"(w367) -> ()
            n295 = local write "Green 2"(w367) -> ()
            n296 = local write "Red 2"(w367) -> ()
            n297 = call-poly <vilib>:"Digital Write.vi"("Error In"=w370, "Output Value"=w367, "DO Channel"=8, "LINX Resource"=w369) -> ()  [unwired: 6 in, 2 out]
            n298 = call-poly <vilib>:"Digital Write.vi"("Error In"=w370, "Output Value"=w368, "DO Channel"=9, "LINX Resource"=w369) -> ()  [unwired: 6 in, 2 out]
            n299 = call-poly <vilib>:"Digital Write.vi"("Error In"=w370, "Output Value"=w367, "DO Channel"=10, "LINX Resource"=w369) -> ()  [unwired: 6 in, 2 out]
            n300 = call-poly <vilib>:"Digital Write.vi"("Error In"=w370, "Output Value"=w367, "DO Channel"=11, "LINX Resource"=w369) -> ()  [unwired: 6 in, 2 out]
            n301 = call-poly <vilib>:"Digital Write.vi"("Error In"=w370, "Output Value"=w368, "DO Channel"=12, "LINX Resource"=w369) -> ()  [unwired: 6 in, 2 out]
            n302 = call-poly <vilib>:"Digital Write.vi"("Error In"=w370, "Output Value"=w367, "DO Channel"=13, "LINX Resource"=w369) -> ()  [unwired: 6 in, 2 out]
          }
          frame #2 {
            n303 = call "Time Delay"() -> ()  [unwired: 11 in, 1 out]
          }
        }
      }
    }
  }
  n304 = while {
    stop <- "Stop" stop-if-true
    w382 = 1
    n305 = Wait (ms)(milliseconds to wait=100) -> ()  [unwired: 1 out]
    n306 = call-poly <vilib>:"Read Delimited Spreadsheet.vi"("file path (dialog if empty)"=path "C:/project/queue_data.txt", "delimiter (\\t)"="," ("delimiter (\\t)")) -> ("first row"=w387:dbl[])  [unwired: 8 in, 5 out]
    n307 = Index Array(array=w387) -> (element #1=w386:dbl, element #2=w385:dbl, element #3=w384:dbl, element #4=w383:dbl)  [unwired: 4 in]
    n308 = Equal?(x=w384, y=w382) -> (x = y?=w378:bool)
    n309 = Equal?(x=w383, y=w382) -> (x = y?=w377:bool)
    n310 = local write "Lane 1 PCE"(w386) -> ()
    n311 = local write "Lane 2 PCE"(w385) -> ()
    n312 = local write "Emergency 2"(w377) -> ()
    n313 = local write "Emergency 1"(w378) -> ()
  }
